vi "labtest.vi"() -> ()   [LabVIEW 2014, in "Files Library.lvlib"]
uses:
  Files Library.lvlib
  Icons/Delete Row Control.ctl
  Icons/Temperature control.ctl
  Icons/Time Limit.ctl
  Icons/speed control.ctl
  Icons/Recipe Control.ctl
  MASTER/MASTER.lvclass
  Global/Recipe download global.vi
  Global/ClockWise Global.vi
panel:
  in  "Tab Control 3":T1(tab)
  out "Direction":string
  out "Time Limit":string
  out "Temperature Limit":string
  out "Speed":string
  in  "Login Password":string
  out "Timer":u16
  out "Current Temperature":u16
  in  "Delete":bool
  in  "Add":bool
  in  "Password List":i32(listbox)
  in  "New Password":string
  in  "Recipe Download":T2
  in  "Speed":T3
  in  "Time Limit":T4
  in  "Temperature":T5
  in  "Delete Row":T6
  in  "Recipe":i32(listbox)
  in  "Delete Recipe":bool
  in  "Add Recipe":bool
  in  "Clockwise/Reverse":bool
  in  "Start":bool
  in  "Exit":bool
  out "User Enable":bool
  out "Admin Enable":bool
  in  "Login":bool
  out "error out":errorcluster
  in  "error in (no error)":errorcluster
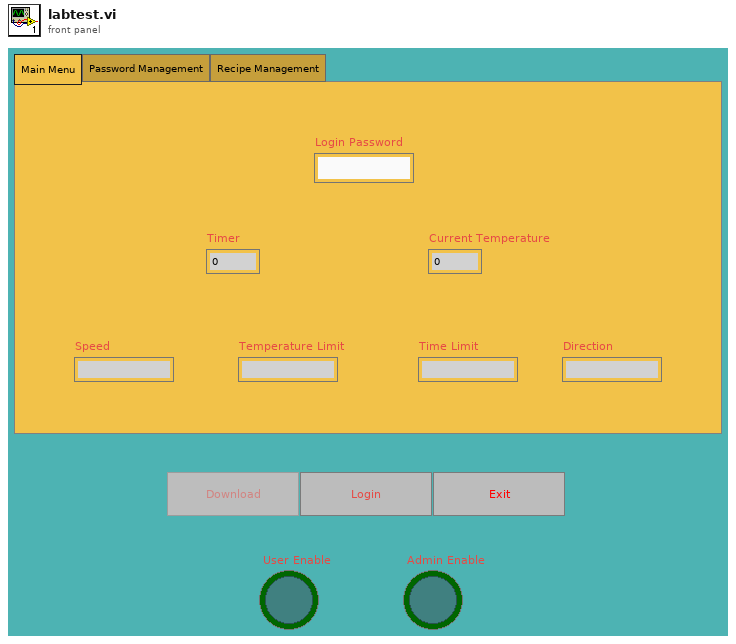
[diagram p1: front panel]
types:
  T1 = enum32{"Main Menu", "Password Management", "Recipe Management"}
  T2 = typedef "Recipe Control.ctl" = u16
  T3 = typedef "speed control.ctl" = u16
  T4 = typedef "Time Limit.ctl" = u16
  T5 = typedef "Temperature control.ctl" = u16
  T6 = typedef "Delete Row Control.ctl" = u16
  T7 = enum8{"Enabled", "Disabled", "Disabled and Grayed Out"}
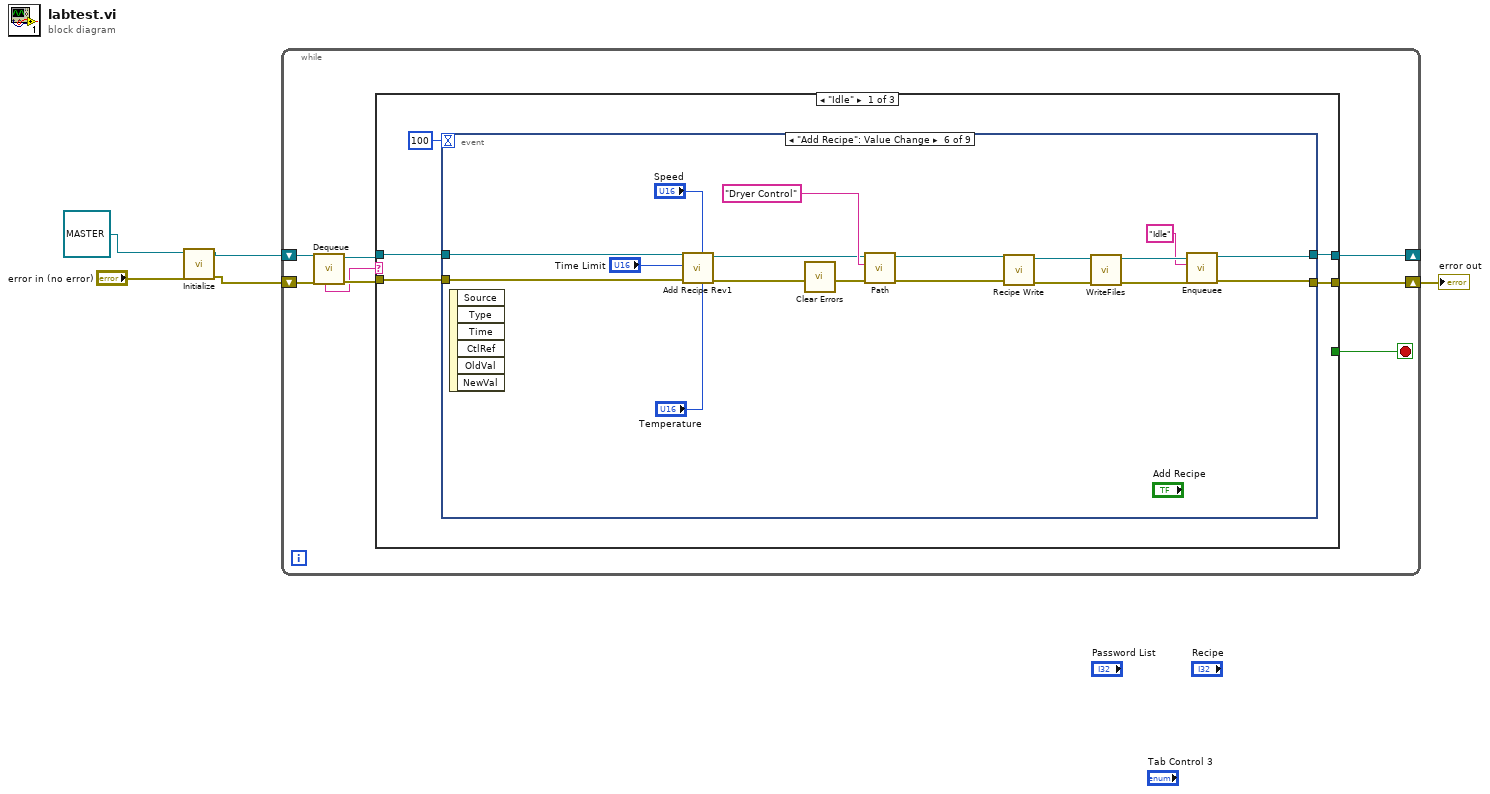
[diagram p0: block diagram]
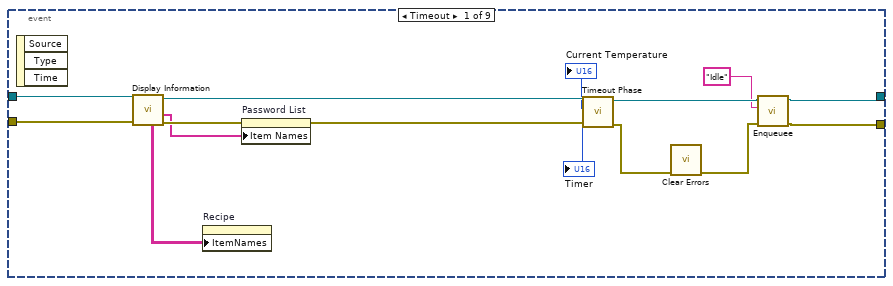
[diagram p2: hidden frame]
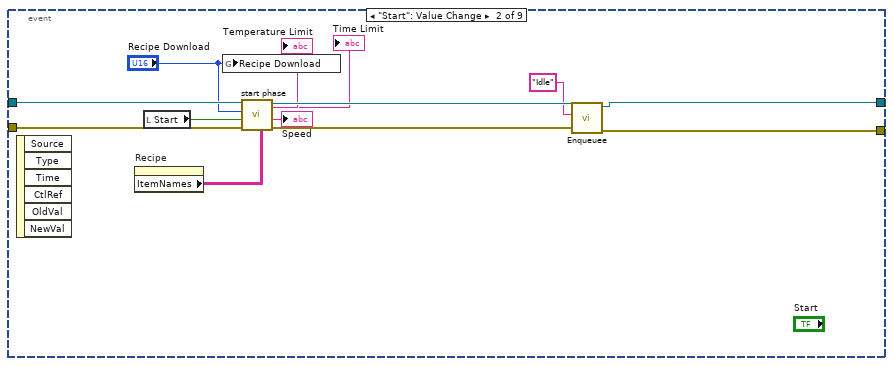
[diagram p3: hidden frame]
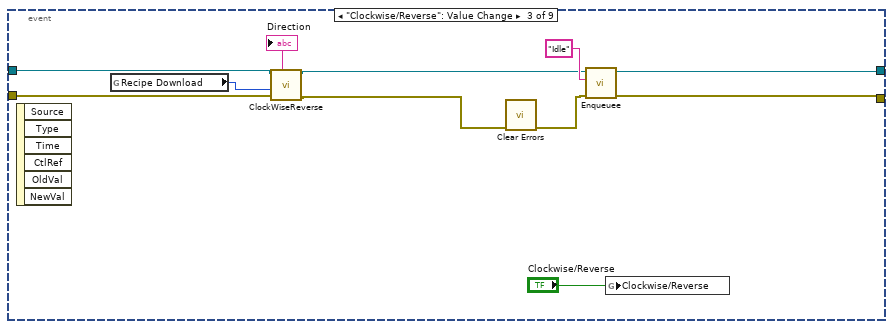
[diagram p4: hidden frame]
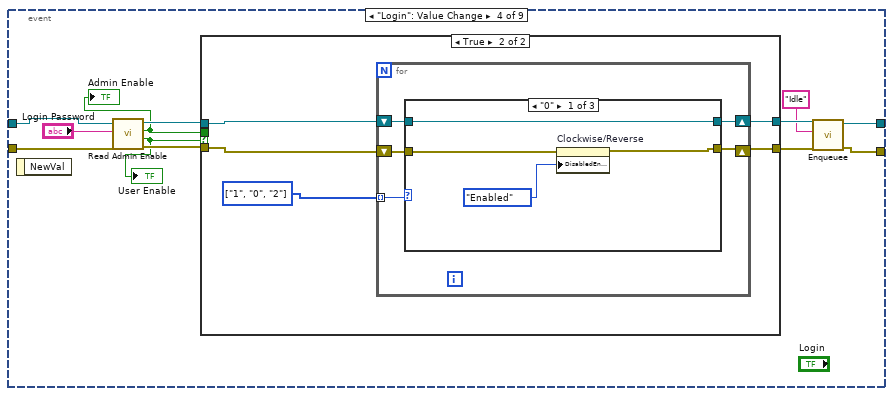
[diagram p5: hidden frame]
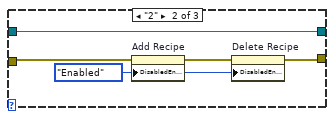
[diagram p7: hidden frame]
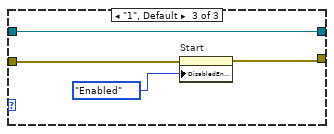
[diagram p8: hidden frame]
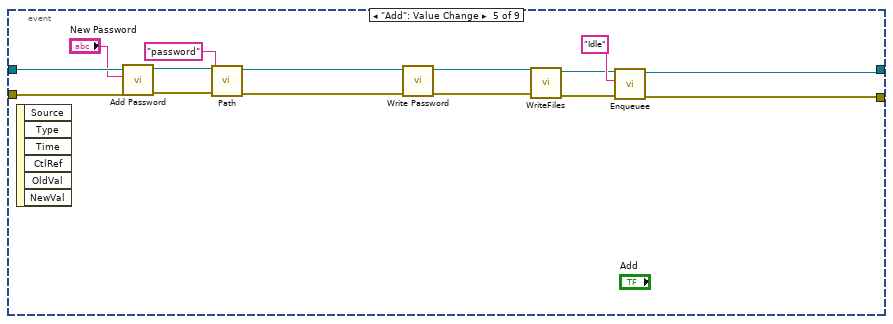
[diagram p9: hidden frame]
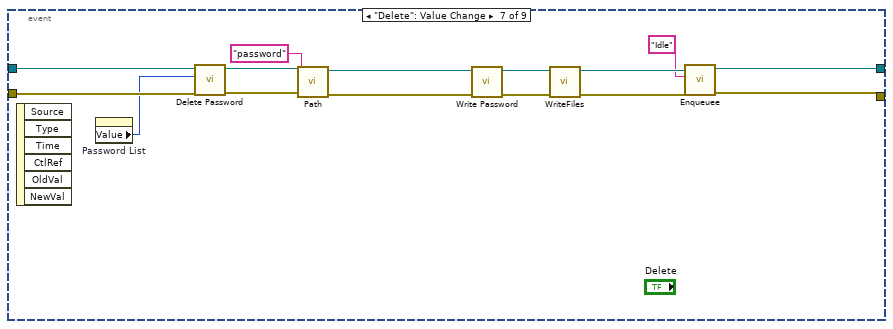
[diagram p10: hidden frame]
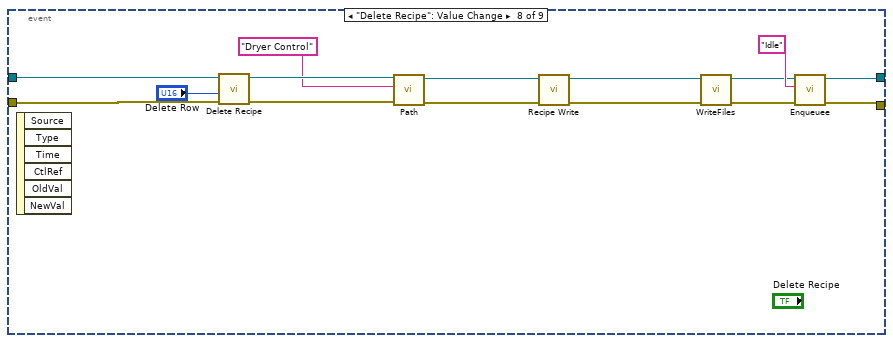
[diagram p11: hidden frame]
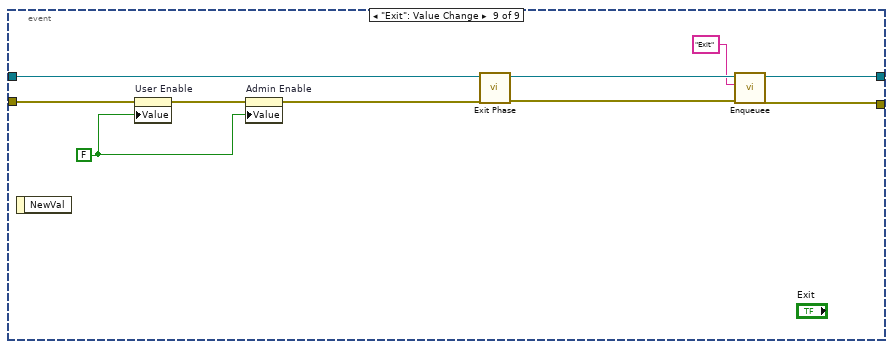
[diagram p12: hidden frame]
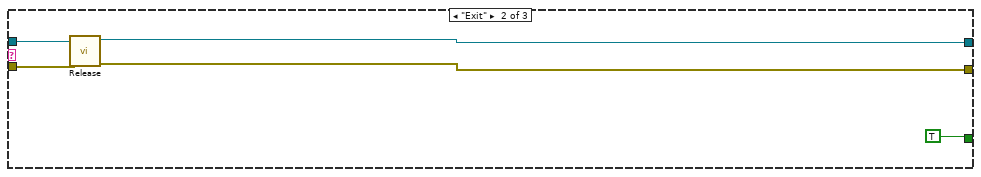
[diagram p13: hidden frame]
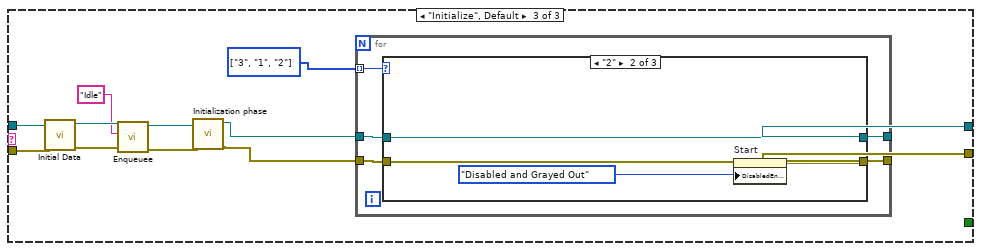
[diagram p14: hidden frame]
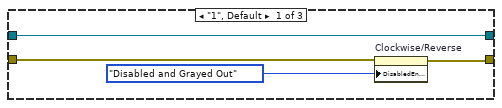
[diagram p15: hidden frame]
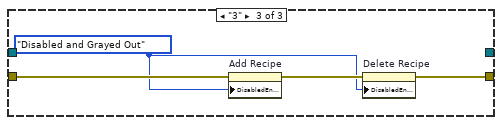
[diagram p16: hidden frame]
diagram:
  n1 = call-dynamic "Initialize.vi"("error in (no error)"="error in (no error)", "MASTER in"=refnum<class "MASTER.lvclass"> refnum ("Files Library.lvlib:MASTER.lvclass")) -> ("error out"=w1:errorcluster, "MASTER out"=w2:refnum<class "MASTER.lvclass">)  [unwired: 8 in]
  n2 = while {
    shift-right: [w13] -> _
    shift-left: w2 -> [w10]
    shift-right: [w12] -> w5
    shift-left: w1 -> [w9]
    stop <- w11 stop-if-true
    n3 = call-dynamic "Dequeue.vi"("error in (no error)"=w9, "MASTER in"=w10) -> ("error out"=w7:errorcluster, "MASTER out"=w8:refnum<class "MASTER.lvclass">, "state"=w6:string)  [unwired: 7 in]
    n4 = case shown="\"Idle\"" w6 {
      tunnel: w8 -> [w18 w169 w180]
      tunnel: w7 -> [w17 w168 w179]
      tunnel: [w16 w171 w183] -> w13
      tunnel: [w15 w170 w182] -> w12
      tunnel: [_ TRUE _] -> w11
      frame "Idle" {
        n5 = event shown="[5] \"Add Recipe\": Value Change" {
          selector: _ -> [_ _ _ _ _ _ _ _ _]
          dyn-events: _ -> [_ _ _ _ _ _ _ _ _]
          timeout: 100 -> [_ _ _ _ _ _ _ _ _]
          tunnel: w18 -> [w32 w44 w52 w68 w109 w120 w142 w152 w167]
          tunnel: w17 -> [w31 w46 w51 w69 w108 w119 w141 w151 w161]
          tunnel: [w26 w40 w57 w60 w97 w127 w130 w157 w163] -> w16
          tunnel: [w25 w39 w56 w59 w96 w126 w129 w156 w162] -> w15
          event Timeout {
            n6 = event-data() -> ()  [unwired: 1 in, 3 out]
            n7 = call-dynamic "Display Information.vi"("error in (no error)"=w31, "Master in"=w32) -> ("error out"=w30:errorcluster, "Passwords"=w21:string[], "Master out"=w29:refnum<class "MASTER.lvclass">, "Recipe Indicator"=w24:string[][])  [unwired: 5 in, 1 out]
            n8 = property on="Recipe" class="MCListbox (strict)"("ItemNames"=w24) -> ()  [unwired: 2 in, 2 out]
            n9 = property on="Password List" class="LstBox (strict)"(error in=w30, "Item Names"=w21) -> (error out=w33:errorcluster)  [unwired: 1 in, 1 out]
            n10 = call-dynamic "Timeout Phase.vi"("error in (no error)"=w33, "Programming Logic in"=w29) -> ("error out"=w23:errorcluster, "Programming Logic out"=w28:refnum<class "MASTER.lvclass">, "Timer"=→"Timer":u16, "Temperature"=→"Current Temperature":u16)  [unwired: 6 in]
            n11 = call <vilib>:"Clear Errors.vi"("error in (no error)"=w23) -> ("error out"=w22:errorcluster)  [unwired: 5 in, 1 out]
            n12 = call-dynamic "Enqueuee.vi"("error in (no error)"=w22, "State"="Idle", "MASTER in"=w28) -> ("error out"=w25:errorcluster, "MASTER out"=w26:refnum<class "MASTER.lvclass">)  [unwired: 7 in]
          }
          event "Start": Value Change {
            n13 = event-data() -> ()  [unwired: 1 in, 6 out]
            n14 = property on="Recipe" class="MCListbox (strict)"() -> ("ItemNames"=w38:string[][])  [unwired: 2 in, 2 out]
            n15 = local read "Start"() -> (w45:bool)
            n16 = global write "Recipe download global.vi" "Recipe Download"("Recipe Download") -> ()
            n17 = call-dynamic "start phase.vi"("array"=w38, "error in (no error)"=w46, "Start"=w45, "index (row)"="Recipe Download", "Programming Logic in"=w44) -> ("error out"=w42:errorcluster, "Speed"=→"Speed":string, "Programming Logic out"=w43:refnum<class "MASTER.lvclass">, "Temp"=→"Temperature Limit":string, "Time"=→"Time Limit":string)  [unwired: 2 in]
            n18 = call-dynamic "Enqueuee.vi"("error in (no error)"=w42, "State"="Idle", "MASTER in"=w43) -> ("error out"=w39:errorcluster, "MASTER out"=w40:refnum<class "MASTER.lvclass">)  [unwired: 7 in]
          }
          event "Clockwise/Reverse": Value Change {
            n19 = event-data() -> ()  [unwired: 1 in, 6 out]
            n20 = global read "Recipe download global.vi" "Recipe Download"() -> (w48:u16)
            n21 = call "ClockWiseReverse.vi"("error in (no error)"=w51, "index (row)"=w48, "Programming Logic in"=w52) -> ("error out"=w49:errorcluster, "Programming Logic out"=w50:refnum<class "MASTER.lvclass">, "Direction"=→"Direction":string)  [unwired: 6 in]
            n22 = call <vilib>:"Clear Errors.vi"("error in (no error)"=w49) -> ("error out"=w54:errorcluster)  [unwired: 5 in, 1 out]
            n23 = call-dynamic "Enqueuee.vi"("error in (no error)"=w54, "State"="Idle", "MASTER in"=w50) -> ("error out"=w56:errorcluster, "MASTER out"=w57:refnum<class "MASTER.lvclass">)  [unwired: 7 in]
            n24 = global write "ClockWise Global.vi" "Clockwise/Reverse"("Clockwise/Reverse") -> ()
          }
          event "Login": Value Change {
            n25 = event-data() -> ()  [unwired: 1 in, 1 out]
            n26 = call-dynamic "Read Admin Enable.vi"("error in (no error)"=w69, "Login PWD"="Login Password", "Master in"=w68) -> ("error out"=w65:errorcluster, "User Enable"=w64:bool, "Admin Enable"=w63:bool, "Master out"=w66:refnum<class "MASTER.lvclass">)  [unwired: 5 in]
            "Admin Enable" <- w63
            "User Enable" <- w64
            n27 = case shown="True" w64 {
              tunnel: w63 -> [_ _]
              tunnel: w65 -> [w70 w76]
              tunnel: w66 -> [w71 w74]
              tunnel: [w70 w75] -> w61
              tunnel: [w71 w73] -> w62
              frame False {
              }
              frame True {
                w72 = enum16{"2", "1", "0"}[] [enum."1", enum."0", enum."2"] items=["2", "1", "0"]
                n28 = for {
                  shift-right: [w78] -> w73
                  shift-left: w74 -> [w79]
                  shift-right: [w80] -> w75
                  shift-left: w76 -> [w81]
                  tunnel: w72 -> [w77] mode=indexing
                  n29 = case shown="\"0\"" w77 {
                    tunnel: w81 -> [w85 w88 w93]
                    tunnel: [w82 w90 w92] -> w80
                    tunnel: w79 -> [w84 w86 w94]
                    tunnel: [w84 w86 w94] -> w78
                    frame "0" {
                      n30 = property on="Clockwise/Reverse" class="Bool (strict)"(error in=w85, "DisabledEnum"=T7."Enabled" ("Disabled")) -> (error out=w82:errorcluster)  [unwired: 1 in, 1 out]
                    }
                    frame "2" {
                      w87 = T7."Enabled" ("Disabled")
                      n31 = property on="Add Recipe" class="Bool"(error in=w88, "DisabledEnum"=w87) -> (error out=w89:errorcluster)  [unwired: 1 in, 1 out]
                      n32 = property on="Delete Recipe" class="Bool"(error in=w89, "DisabledEnum"=w87) -> (error out=w90:errorcluster)  [unwired: 1 in, 1 out]
                    }
                    frame "1", Default {
                      n33 = property on="Start" class="Bool (strict)"(error in=w93, "DisabledEnum"=T7."Enabled" ("Disabled")) -> (error out=w92:errorcluster)  [unwired: 1 in, 1 out]
                    }
                  }
                }
              }
            }
            n34 = call-dynamic "Enqueuee.vi"("error in (no error)"=w61, "State"="Idle", "MASTER in"=w62) -> ("error out"=w59:errorcluster, "MASTER out"=w60:refnum<class "MASTER.lvclass">)  [unwired: 7 in]
          }
          event "Add": Value Change {
            n35 = event-data() -> ()  [unwired: 1 in, 6 out]
            n36 = call-dynamic "Add Password.vi"("error in (no error)"=w108, "Write Password"="New Password", "Master in"=w109) -> ("error out"=w104:errorcluster, "Master out"=w105:refnum<class "MASTER.lvclass">)  [unwired: 7 in]
            n37 = call-dynamic "Path.vi"("error in (no error)"=w104, "pathname"="password", "Master in"=w105) -> ("error out"=w102:errorcluster, "Master out"=w103:refnum<class "MASTER.lvclass">)  [unwired: 7 in]
            n38 = call-dynamic "Write Password.vi"("error in (no error)"=w102, "Master in"=w103) -> ("error out"=w100:errorcluster, "Master out"=w101:refnum<class "MASTER.lvclass">)  [unwired: 8 in]
            n39 = call-dynamic "WriteFiles.vi"("error in (no error)"=w100, "Master in"=w101) -> ("error out"=w98:errorcluster, "Master out"=w99:refnum<class "MASTER.lvclass">)  [unwired: 8 in]
            n40 = call-dynamic "Enqueuee.vi"("error in (no error)"=w98, "State"="Idle", "MASTER in"=w99) -> ("error out"=w96:errorcluster, "MASTER out"=w97:refnum<class "MASTER.lvclass">)  [unwired: 7 in]
          }
          event "Add Recipe": Value Change {
            n41 = event-data() -> ()  [unwired: 1 in, 6 out]
            n42 = call-dynamic "Add Recipe Rev1.vi"("Temperature"="Temperature", "Speed"="Speed", "error in (no error)"=w119, "Time Limit"="Time Limit", "MASTER in"=w120) -> ("error out"=w117:errorcluster, "MASTER out"=w118:refnum<class "MASTER.lvclass">)  [unwired: 5 in]
            n43 = call <vilib>:"Clear Errors.vi"("error in (no error)"=w117) -> ("error out"=w122:errorcluster)  [unwired: 5 in, 1 out]
            n44 = call-dynamic "Path.vi"("error in (no error)"=w122, "pathname"="Dryer Control", "Master in"=w118) -> ("error out"=w113:errorcluster, "Master out"=w116:refnum<class "MASTER.lvclass">)  [unwired: 7 in]
            n45 = call-dynamic "Recipe Write.vi"("error in (no error)"=w113, "MASTER in"=w116) -> ("error out"=w114:errorcluster, "MASTER out"=w115:refnum<class "MASTER.lvclass">)  [unwired: 8 in]
            n46 = call-dynamic "WriteFiles.vi"("error in (no error)"=w114, "Master in"=w115) -> ("error out"=w124:errorcluster, "Master out"=w125:refnum<class "MASTER.lvclass">)  [unwired: 8 in]
            n47 = call-dynamic "Enqueuee.vi"("error in (no error)"=w124, "State"="Idle", "MASTER in"=w125) -> ("error out"=w126:errorcluster, "MASTER out"=w127:refnum<class "MASTER.lvclass">)  [unwired: 7 in]
          }
          event "Delete": Value Change {
            n48 = event-data() -> ()  [unwired: 1 in, 6 out]
            n49 = property on="Password List" class="LstBox (strict)"() -> ("Value"=w133:i32)  [unwired: 2 in, 2 out]
            n50 = call-dynamic "Delete Password.vi"("error in (no error)"=w141, "index"=w133, "Master in"=w142) -> ("error out"=w139:errorcluster, "Master out"=w140:refnum<class "MASTER.lvclass">)  [unwired: 7 in]
            n51 = call-dynamic "Path.vi"("error in (no error)"=w139, "pathname"="password", "Master in"=w140) -> ("error out"=w137:errorcluster, "Master out"=w138:refnum<class "MASTER.lvclass">)  [unwired: 7 in]
            n52 = call-dynamic "Write Password.vi"("error in (no error)"=w137, "Master in"=w138) -> ("error out"=w135:errorcluster, "Master out"=w136:refnum<class "MASTER.lvclass">)  [unwired: 8 in]
            n53 = call-dynamic "WriteFiles.vi"("error in (no error)"=w135, "Master in"=w136) -> ("error out"=w131:errorcluster, "Master out"=w132:refnum<class "MASTER.lvclass">)  [unwired: 8 in]
            n54 = call-dynamic "Enqueuee.vi"("error in (no error)"=w131, "State"="Idle", "MASTER in"=w132) -> ("error out"=w129:errorcluster, "MASTER out"=w130:refnum<class "MASTER.lvclass">)  [unwired: 7 in]
          }
          event "Delete Recipe": Value Change {
            n55 = event-data() -> ()  [unwired: 1 in, 6 out]
            n56 = call-dynamic "Delete Recipe.vi"("error in (no error)"=w151, "Delete Row"="Delete Row", "MASTER in"=w152) -> ("error out"=w149:errorcluster, "MASTER out"=w150:refnum<class "MASTER.lvclass">)  [unwired: 7 in]
            n57 = call-dynamic "Path.vi"("error in (no error)"=w149, "pathname"="Dryer Control", "Master in"=w150) -> ("error out"=w146:errorcluster, "Master out"=w147:refnum<class "MASTER.lvclass">)  [unwired: 7 in]
            n58 = call-dynamic "Recipe Write.vi"("error in (no error)"=w146, "MASTER in"=w147) -> ("error out"=w144:errorcluster, "MASTER out"=w145:refnum<class "MASTER.lvclass">)  [unwired: 8 in]
            n59 = call-dynamic "WriteFiles.vi"("error in (no error)"=w144, "Master in"=w145) -> ("error out"=w153:errorcluster, "Master out"=w154:refnum<class "MASTER.lvclass">)  [unwired: 8 in]
            n60 = call-dynamic "Enqueuee.vi"("error in (no error)"=w153, "State"="Idle", "MASTER in"=w154) -> ("error out"=w156:errorcluster, "MASTER out"=w157:refnum<class "MASTER.lvclass">)  [unwired: 7 in]
          }
          event "Exit": Value Change {
            w158 = FALSE
            n61 = event-data() -> ()  [unwired: 1 in, 1 out]
            n62 = property on="User Enable" class="Bool (strict)"(error in=w161, "Value"=w158) -> (error out=w160:errorcluster)  [unwired: 1 in, 1 out]
            n63 = property on="Admin Enable" class="Bool (strict)"(error in=w160, "Value"=w158) -> (error out=w159:errorcluster)  [unwired: 1 in, 1 out]
            n64 = call-dynamic "Exit Phase.vi"("error in (no error)"=w159, "Programming Logic in"=w167) -> ("error out"=w165:errorcluster, "Programming Logic out"=w166:refnum<class "MASTER.lvclass">)  [unwired: 8 in]
            n65 = call-dynamic "Enqueuee.vi"("error in (no error)"=w165, "State"="Exit", "MASTER in"=w166) -> ("error out"=w162:errorcluster, "MASTER out"=w163:refnum<class "MASTER.lvclass">)  [unwired: 7 in]
          }
        }
      }
      frame "Exit" {
        n66 = call-dynamic "Release.vi"("error in (no error)"=w168, "MASTER in"=w169) -> ("error out"=w170:errorcluster, "MASTER out"=w171:refnum<class "MASTER.lvclass">)  [unwired: 8 in]
      }
      frame "Initialize", Default {
        w184 = enum16{"3", "1", "2"}[] [enum."3", enum."1", enum."2"] items=["3", "1", "2"]
        n67 = call-dynamic "Initial Data.vi"("error in (no error)"=w179, "Master in"=w180) -> ("error out"=w177:errorcluster, "Master out"=w176:refnum<class "MASTER.lvclass">)  [unwired: 8 in]
        n68 = call-dynamic "Enqueuee.vi"("error in (no error)"=w177, "State"="Idle", "MASTER in"=w176) -> ("error out"=w173:errorcluster, "MASTER out"=w174:refnum<class "MASTER.lvclass">)  [unwired: 7 in]
        n69 = call-dynamic "Initialization phase.vi"("error in (no error)"=w173, "Programming Logic in"=w174) -> ("error out"=w181:errorcluster, "Programming Logic out"=w178:refnum<class "MASTER.lvclass">)  [unwired: 8 in]
        n70 = for {
          tunnel: w184 -> [w189] mode=indexing
          tunnel: w178 -> [w188]
          tunnel: [w187] -> w183
          tunnel: [w186] -> w182
          tunnel: w181 -> [w185]
          n71 = case shown="\"2\"" w189 {
            tunnel: w188 -> [w193 w197 _]
            tunnel: [w193 w197 _] -> w187
            tunnel: [w191 w196 w199] -> w186
            tunnel: w185 -> [w192 w194 w201]
            frame "1", Default {
              n72 = property on="Clockwise/Reverse" class="Bool (strict)"(error in=w192, "DisabledEnum"=T7."Disabled and Grayed Out" ("Disabled")) -> (error out=w191:errorcluster)  [unwired: 1 in, 1 out]
            }
            frame "2" {
              n73 = property on="Start" class="Bool (strict)"(error in=w194, "DisabledEnum"=T7."Disabled and Grayed Out" ("Disabled")) -> (error out=w196:errorcluster)  [unwired: 1 in, 1 out]
            }
            frame "3" {
              w198 = T7."Disabled and Grayed Out" ("Disabled")
              n74 = property on="Add Recipe" class="Bool"(error in=w201, "DisabledEnum"=w198) -> (error out=w200:errorcluster)  [unwired: 1 in, 1 out]
              n75 = property on="Delete Recipe" class="Bool"(error in=w200, "DisabledEnum"=w198) -> (error out=w199:errorcluster)  [unwired: 1 in, 1 out]
            }
          }
        }
      }
    }
  }
  "error out" <- w5
